vi "GetBinaryData.vi"(8 "error in (no error)":errorcluster, 11 "SettingsFile in":refnum<class "SettingsFile.lvclass">) -> (0 "error out":errorcluster, 1 "HaveData":bool, 2 "BinaryData":string, 3 "SettingsFile out":refnum<class "SettingsFile.lvclass">)   [LabVIEW 2018, in "SettingsFile.lvclass"]
uses:
  SettingsFile.lvclass
  SettingsFile.lvclass/SettingsFile.ctl
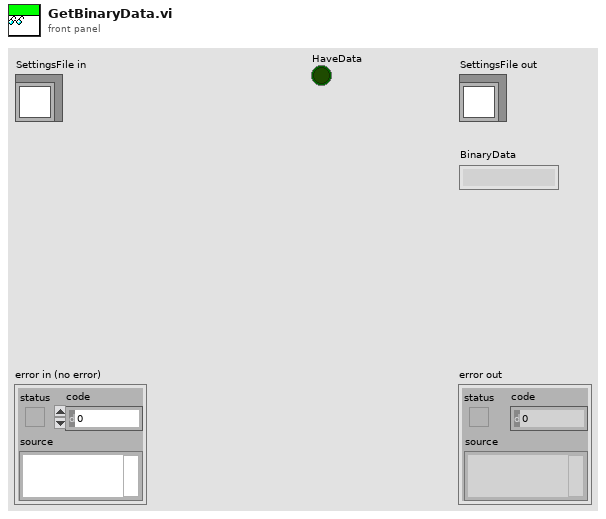
[diagram p1: front panel]
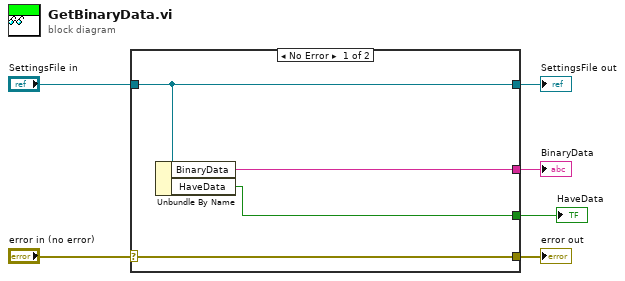
[diagram p0: block diagram]
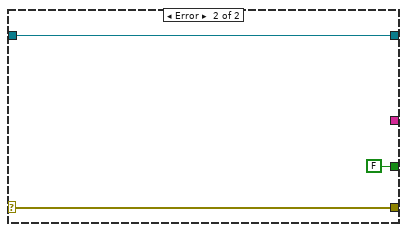
[diagram p2: hidden frame]
diagram:
  n1 = case shown="No Error" "error in (no error)" {
    selector: "error in (no error)" -> [w10 w12]
    tunnel: [w10 w12] -> w5
    tunnel: [w9 w13] -> w3
    tunnel: "SettingsFile in" -> [w9 w13]
    tunnel: [w8 _] -> w2
    tunnel: [w7 FALSE ("HaveData")] -> w1
    frame No Error {
      n2 = Unbundle By Name(w9) -> ("BinaryData"=w8:string, "HaveData"=w7:bool)
    }
    frame Error {
    }
  }
  "error out" <- w5
  "SettingsFile out" <- w3
  "BinaryData" <- w2
  "HaveData" <- w1
